vi "Config.vi"(8 "error in (no error)":errorcluster, 10 "Setting":variant, 11 "Keysight 6700C in":refnum<class "Keysight 6700C.lvclass">) -> (0 "error out":errorcluster, 3 "Keysight 6700C out":refnum<class "Keysight 6700C.lvclass">)   [LabVIEW 2025, in "Power Supply.lvlib" / "Keysight 6700C.lvclass"]
uses:
  Keysight 6700C.lvclass
  Keysight 6700C.lvclass/Keysight 6700C.ctl
  <instrlib>/Agilent N6700 Series/Agilent N6700 Series.lvlib
  PS Channel/Power Supply Channel.lvclass
  PS Channel configuration/Power Supply Channel configuration.lvclass
  Users/Public/Documents/Sandia National Labs/TSS Plugin/Abstract Engine.lvlibp/Plugin/Abstract/Abstract Instrument/Channel.ctl
  Users/Public/Documents/Sandia National Labs/TSS Plugin/Abstract Engine.lvlibp/Plugin/Abstract/Abstract Instrument/Abstract Instrument.lvclass
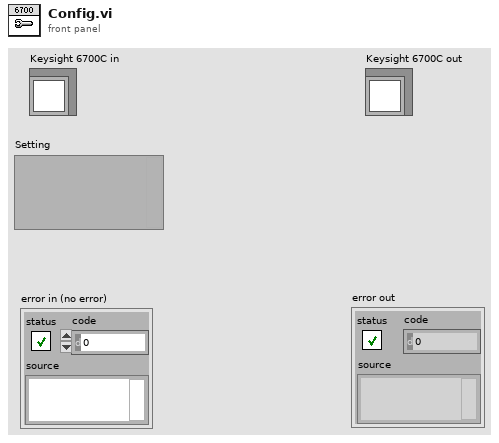
[diagram p1: front panel]
types:
  T1 = typedef "Abstract Engine.lvlibp/Abstract Instrument.lvclass/Channel.ctl" = cluster{"Alias":string, "DataType":enum16{"Anaolg Input", "Waveform"}, "Unit":enum16{"---", "V", "A", "Ohm", "Hz", "uF", "degC", "deg"}, "Upper limit":dbl, "Lower limit":dbl, "Measurement":variant}
  T2 = typedef "Power Supply.lvlib/Power Supply Channel configuration.lvclass/PS Channel Setting.ctl" = cluster{"Driver":string, "Pin":string, "Test Voltage":string, "Voltage Low":dbl, "Voltage Norminal":dbl, "Voltage High":dbl, "PreTest Voltage":dbl, "PreTest Current":dbl, "Current Limit":dbl}
  T3 = typedef "Abstract Engine.lvlibp/Channel configuration.lvclass/Default Channel.ctl" = cluster{"Address":string, "SW Alias":string, "Enabled":bool, "Type":string, "Description":string}
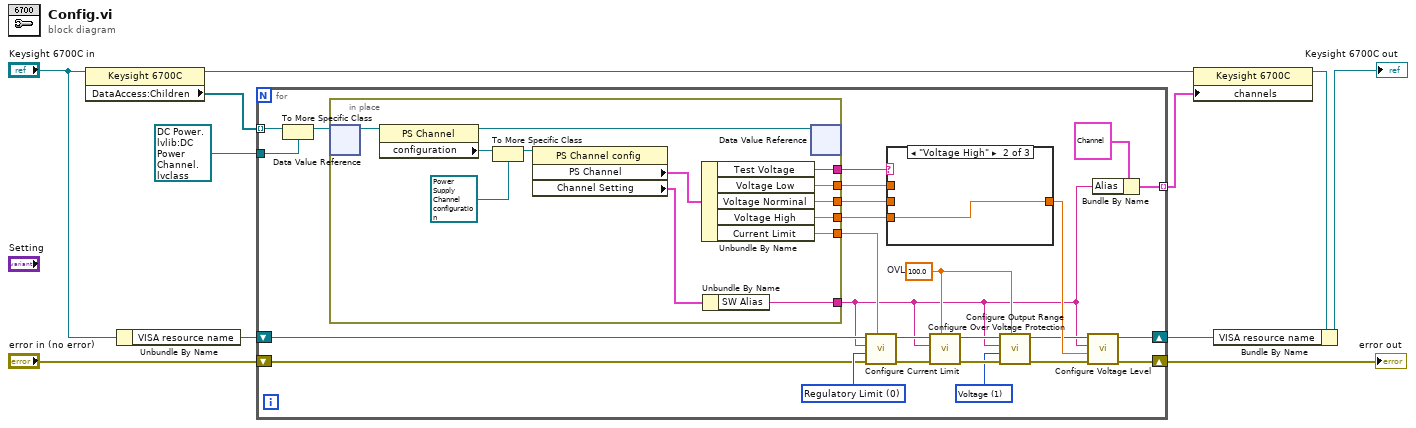
[diagram p0: block diagram]
diagram:
  n1 = property class="Keysight 6700C"(reference="Keysight 6700C in") -> (reference out=w5:refnum<class "Keysight 6700C.lvclass">, "DataAccess:Children"=w4:refnum<data-value>[])  [unwired: 1 in, 1 out]
  n2 = Unbundle By Name("Keysight 6700C in") -> ("VISA resource name"=w9:refnum<visa-resource-name>)
  n3 = for {
    shift-right: [w31] -> w8
    shift-left: w9 -> [w24]
    shift-right: [w36] -> w11
    shift-left: "error in (no error)" -> [w26]
    tunnel: w4 -> [w30] mode=indexing
    tunnel: refnum<data-value> refnum ("data value reference") -> [w29]
    tunnel: [w13] -> w1 mode=indexing
    w21 = 100.0  # OVL
    w32 = 1 items=["Voltage"=1, "Current"=0] ("Range Type (1: Voltage)")
    w35 = 0 items=["Regulatory Limit", "Trip Limit"] ("Behavior (0: Regulatory Limit)")
    n4 = To More Specific Class(target class=w29, reference=w30) -> (specific class reference=w28:refnum<data-value>)  [unwired: 1 in, 1 out]
    n5 = in-place {
      in-place-border: [w42] -> w14
      in-place-border: [w41] -> w22
      in-place-border: [w40] -> w20
      in-place-border: [w39] -> w19
      in-place-border: [w38] -> w18
      in-place-border: [w37] -> w17
      # "Initialize the front panel controls when loaded"
      n6 = in-place-dvr #1(w28) -> (w49:refnum<class "Power Supply Channel.lvclass">)  [unwired: 1 out]
      n7 = property class="PS Channel"(reference=w49) -> (reference out=w48:refnum<class "Power Supply Channel.lvclass">, "configuration"=w47:refnum<class "CEF_serializable configuration.lvclass">)  [unwired: 1 in, 1 out]
      n8 = To More Specific Class(target class=refnum<class "Power Supply Channel configuration.lvclass"> refnum ("DC Power.lvlib:DCPower Channel configuration.lvclass"), reference=w47) -> (specific class reference=w46:refnum<class "Power Supply Channel configuration.lvclass">)  [unwired: 1 in, 1 out]
      n9 = property class="PS Channel config"(reference=w46) -> ("PS Channel"=w44:T2, "Channel Setting"=w43:T3)  [unwired: 1 in, 2 out]
      n10 = Unbundle By Name(w44) -> ("Test Voltage"=w40:string, "Voltage Low"=w39:dbl, "Voltage Norminal"=w38:dbl, "Voltage High"=w37:dbl, "Current Limit"=w41:dbl)
      n11 = Unbundle By Name(w43) -> ("SW Alias"=w42:string)
      n12 = in-place-dvr #1(w48) -> ()  [unwired: 2 out]
    }
    n13 = call <instrlib>:"Configure Current Limit.vi"("Limit (0.0 amps)"=w22, "error in (no error)"=w26, "Behavior (0: Regulatory Limit)"=w35, "Channel Name (1)"=w14, "VISA resource name"=w24) -> ("error out"=w25:errorcluster, "VISA resource name out"=w23:refnum<visa-resource-name>)  [unwired: 5 in]
    n14 = case shown="\"Voltage High\"" w20 {
      tunnel: w19 -> [_ _ w52]
      tunnel: w18 -> [w50 _ _]
      tunnel: w17 -> [_ w51 _]
      tunnel: [w50 w51 w52] -> w27
      frame "Voltage Norminal", Default {
      }
      frame "Voltage High" {
      }
      frame "Voltage Low" {
      }
    }
    n15 = call <instrlib>:"Configure Over Voltage Protection.vi"("Limit (0.0 volts)"=w21, "error in (no error)"=w25, "Channel Name (1)"=w14, "VISA resource name"=w23) -> ("error out"=w34:errorcluster, "VISA resource name out"=w33:refnum<visa-resource-name>)  [unwired: 6 in]
    n16 = call <instrlib>:"Configure Output Range.vi"("Range (0.0)"=w21, "error in (no error)"=w34, "Range Type (1: Voltage)"=w32, "Channel Name (1)"=w14, "VISA resource name"=w33) -> ("error out"=w16:errorcluster, "VISA resource name out"=w15:refnum<visa-resource-name>)  [unwired: 5 in]
    n17 = call <instrlib>:"Configure Voltage Level.vi"("error in (no error)"=w16, "Level  (0.0 volts)"=w27, "Channel Name (1)"=w14, "VISA resource name"=w15) -> ("error out"=w36:errorcluster, "VISA resource name out"=w31:refnum<visa-resource-name>)  [unwired: 6 in]
    n18 = Bundle By Name(cluster=T1 {"Alias"="ch0", "DataType"=enum."Anaolg Input", "Unit"=enum."V", "Upper limit"=10.0, "Lower limit"=-10.0, "Measurement"=variant} ("Channel"), "Alias"=w14) -> (w13:T1)
  }
  "error out" <- w11
  n19 = property class="Keysight 6700C"(reference=w5, "channels"=w1) -> (reference out=w2:refnum<class "Keysight 6700C.lvclass">)  [unwired: 1 in, 1 out]
  n20 = Bundle By Name(cluster=w2, "VISA resource name"=w8) -> (→"Keysight 6700C out":refnum<class "Keysight 6700C.lvclass">)
